vi "ESP301 Goto.vi"(5 "Axe Inv":bool, 6 "Input Units":i8(ring) items=["mm", "ps"], 7 "ESP301Ref":T1, 8 "error in":errorcluster, 9 "Axis":i8(ring)=1 items=["Axis 1"=1, "Axis 2"=2, "Axis 3"=3], 10 "Position":dbl=0.5, 11 "VISA Rsrc":refnum<visa-resource-name>="GPIB0::7::INSTR") -> (0 "error out":errorcluster, 1 "HighLim":bool, 2 "Pos Out":dbl=0.5, 3 "Warning":bool, 4 "LowLim":bool)   [LabVIEW 2019]
uses:
  <userlib>/ESP300/ESP300 GotoState.ctl
panel:
  out "Move Done":bool
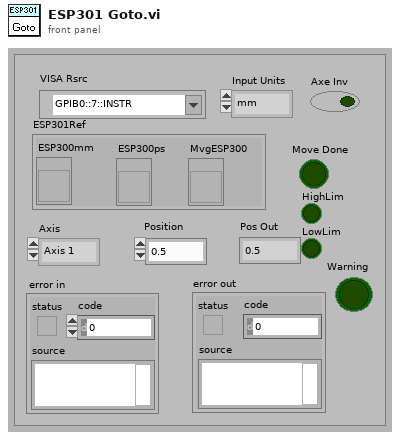
[diagram p1: front panel]
types:
  T1 = cluster{"ESP300mm":refnum<vi>, "ESP300ps":refnum<vi>, "MvgESP300":refnum<vi>}
  T2 = typedef "ESP300 GotoState.ctl" = enum16{"send command", "read position", "check status", "end"}
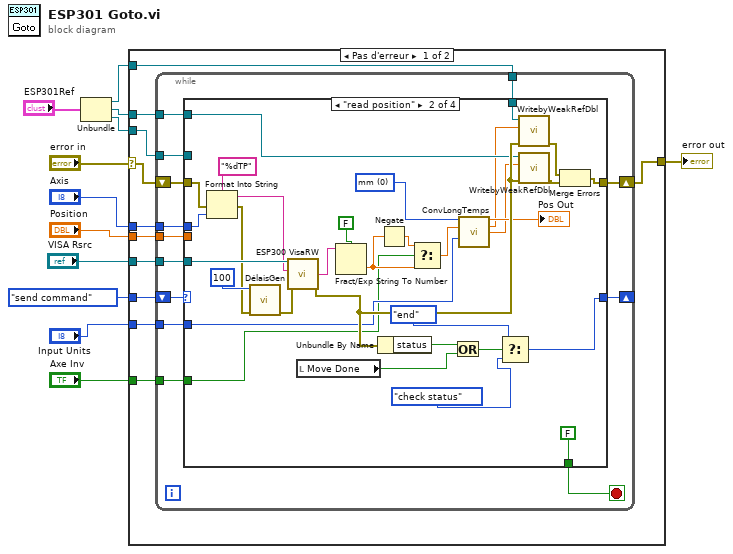
[diagram p0: block diagram]
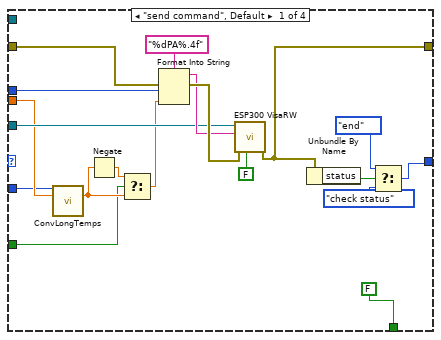
[diagram p2: hidden frame]
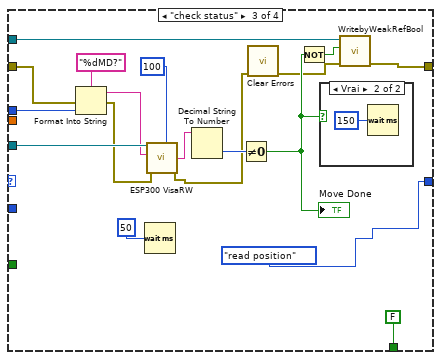
[diagram p3: hidden frame]
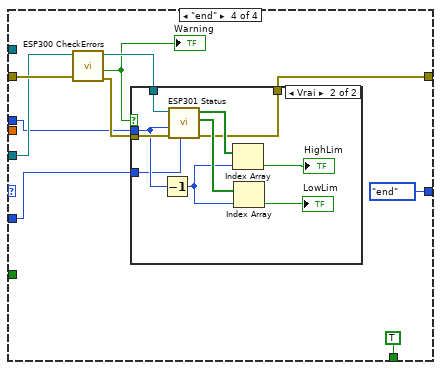
[diagram p5: hidden frame]
diagram:
  n1 = Unbundle("ESP301Ref") -> ("ESP300mm"=w2:refnum<vi>, "ESP300ps"=w4:refnum<vi>, "MvgESP300"=w3:refnum<vi>)
  n2 = case shown="Pas d'erreur" "error in" {
    selector: "error in" -> [w20 w128]
    tunnel: "Axis" -> [w22 _]
    tunnel: "Position" -> [w23 _]
    tunnel: [w19 w128] -> w9
    tunnel: ESP300_GotoState."send command" ("Énum") -> [w21 _]
    tunnel: "VISA Rsrc" -> [w18 _]
    tunnel: w3 -> [w17 _]
    tunnel: "Input Units" -> [w16 _]
    tunnel: w2 -> [w15 _]
    tunnel: w4 -> [w14 _]
    tunnel: "Axe Inv" -> [w13 _]
    frame No Error {
      n3 = while {
        tunnel: w23 -> [w36]
        tunnel: w22 -> [w35]
        shift-right: [w31] -> w19
        shift-left: w20 -> [w33]
        tunnel: w18 -> [w32]
        shift-right: [w29] -> _
        shift-left: w21 -> [w34]
        tunnel: w17 -> [w28]
        tunnel: w16 -> [w27]
        tunnel: w15 -> [w26]
        tunnel: w14 -> [w25]
        tunnel: w13 -> [w24]
        stop <- w30 stop-if-true
        n4 = case shown="\"read position\"" w34 {
          tunnel: w36 -> [w42 _ _ _]
          tunnel: w35 -> [w54 w85 w103 w108]
          tunnel: w33 -> [w53 w84 w102 w114]
          tunnel: w32 -> [w50 w87 w105 w113]
          tunnel: [w47 w68 w90 w109] -> w31
          tunnel: [FALSE FALSE FALSE TRUE] -> w30
          tunnel: [w44 w77 ESP300_GotoState."read position" ("Énum") ESP300_GotoState."end" ("Énum")] -> w29
          tunnel: w28 -> [_ _ w88 _]
          tunnel: w27 -> [w41 w60 _ w107]
          tunnel: w26 -> [_ w66 _ _]
          tunnel: w25 -> [_ w65 _ _]
          tunnel: w24 -> [w37 w56 _ _]
          frame "send command", Default {
            n5 = call <userlib>:"ConvLongTemps.vi"("Input Units"=w41, "Units Input"=w42) -> ("Units mm"=w38:dbl)  [unwired: 10 in, 3 out]
            n6 = Negate(x=w38) -> (-x=w39:dbl)
            n7 = Select(t=w39, s=w37, f=w38) -> (s? t:f=w40:dbl)
            n8 = Format Into String(format string="%dPA%.4f", error in=w53, w54, w40) -> (resulting string=w51:string, error out=w52:errorcluster)  [unwired: 1 in]
            n9 = call <userlib>:"ESP300 VisaRW.vi"("Lecture?(T)"=FALSE, "error in (no error)"=w52, "ChaineCom"=w51, "VISA Rsrc"=w50) -> ("error out"=w47:errorcluster)  [unwired: 3 in, 3 out]
            n10 = Unbundle By Name(w47) -> ("status"=w46:bool)
            n11 = Select(t=ESP300_GotoState."end" ("Énum"), s=w46, f=ESP300_GotoState."check status" ("Énum")) -> (s? t:f=w44:T2)
          }
          frame "read position" {
            w64 = i8 0 items=["mm", "ps"] ("Input Units")
            n12 = Format Into String(format string="%dTP", error in=w84, w85) -> (resulting string=w83:string, error out=w72:errorcluster)  [unwired: 1 in]
            n13 = call "DélaisGen.vi"("error in (no error)"=w72, "ms To Wait"=u32 100 ("milliseconds to wait")) -> ("error out"=w73:errorcluster)  [unwired: 9 in]
            n14 = call <userlib>:"ESP300 VisaRW.vi"("error in (no error)"=w73, "ChaineCom"=w83, "VISA Rsrc"=w87) -> ("error out"=w69:errorcluster, "ChaineRep"=w82:string)  [unwired: 4 in, 2 out]
            n15 = local read "Move Done"() -> (w71:bool)
            n16 = Fract/Exp String To Number(use system decimal point (T)=FALSE ("utiliser le séparateur décimal du système (V)"), string=w82) -> (number=w58:dbl)  [unwired: 2 in, 1 out]
            n17 = Unbundle By Name(w69) -> ("status"=w76:bool)
            n18 = Negate(x=w58) -> (-x=w59:dbl)
            n19 = Select(t=w59, s=w56, f=w58) -> (s? t:f=w57:dbl)
            n20 = Or(x=w76, y=w71) -> (x .or. y?=w75:bool)
            n21 = call <userlib>:"ConvLongTemps.vi"("Input Units"=w64, "Units Input"=w57, "Output Units"=w60) -> ("Units Output"=→"Pos Out":dbl, "Units mm"=w62:dbl, "Units ps"=w61:dbl)  [unwired: 9 in, 1 out]
            n22 = Select(t=ESP300_GotoState."end" ("Énum"), s=w75, f=ESP300_GotoState."check status" ("Énum")) -> (s? t:f=w77:T2)
            n23 = call <userlib>:"WritebyWeakRefDbl.vi"("error in"=w69, "Valeur"=w62, "Control Ref"=w66) -> ("error out"=w67:errorcluster)  [unwired: 8 in]
            n24 = call <userlib>:"WritebyWeakRefDbl.vi"("error in"=w69, "Valeur"=w61, "Control Ref"=w65) -> ("error out"=w70:errorcluster)  [unwired: 8 in]
            n25 = Merge Errors(w67, w70) -> (w68:errorcluster)
          }
          frame "check status" {
            n26 = Format Into String(format string="%dMD?", error in=w102, w103) -> (resulting string=w100:string, error out=w101:errorcluster)  [unwired: 1 in]
            n27 = Wait (ms)(milliseconds to wait=u32 50 ("attente (ms)")) -> ()  [unwired: 1 out]
            n28 = call <userlib>:"ESP300 VisaRW.vi"("Délais (0 ms)"=u32 100, "error in (no error)"=w101, "ChaineCom"=w100, "VISA Rsrc"=w105) -> ("error out"=w95:errorcluster, "ChaineRep"=w99:string)  [unwired: 3 in, 2 out]
            n29 = Decimal String To Number(string=w99) -> (number=w97:i32)  [unwired: 2 in, 1 out]
            n30 = Not Equal To 0?(x=w97) -> (x != 0?=w94:bool)
            "Move Done" <- w94
            n31 = call <vilib>:"Clear Errors.vi"("error in (no error)"=w95) -> ("error out"=w91:errorcluster)  [unwired: 5 in, 1 out]
            n32 = Not(x=w94) -> (.not. x?=w89:bool)
            n33 = case shown="Vrai" w94 {
              frame False {
              }
              frame True {
                n34 = Wait (ms)(milliseconds to wait=u32 150) -> ()  [unwired: 1 out]
              }
            }
            n35 = call <userlib>:"WritebyWeakRefBool.vi"("error in"=w91, "Valeur"=w89, "Control Ref"=w88) -> ("error out"=w90:errorcluster)  [unwired: 8 in]
          }
          frame "end" {
            n36 = call <userlib>:"ESP300 CheckErrors.vi"("error in (no error)"=w114, "Ressource VISA In"=w113) -> ("error out"=w110:errorcluster, "Warning"=w111:bool, "Ressource VISA Out"=w112:refnum<visa-resource-name>)  [unwired: 4 in, 1 out]
            "Warning" <- w111
            n37 = case shown="Vrai" w111 {
              tunnel: w112 -> [_ w127]
              tunnel: w110 -> [w117 w124]
              tunnel: [w117 w123] -> w109
              tunnel: w108 -> [_ w122]
              tunnel: w107 -> [_ w120]
              frame False {
              }
              frame True {
                n38 = Decrement(x=w122) -> (x-1=w121:i8)
                n39 = call <userlib>:"ESP301 Status.vi"("Input Units"=w120, "error in"=w124, "Axis"=w122, "VISA Rsrc"=w127) -> ("error out"=w123:errorcluster, "Low Limit"=w125:bool[], "High Limit"=w126:bool[])  [unwired: 4 in, 1 out]
                n40 = Index Array(array=w126, index=w121) -> (element=→"HighLim":bool)
                n41 = Index Array(array=w125, index=w121) -> (element=→"LowLim":bool)
              }
            }
          }
        }
      }
    }
    frame Error {
    }
  }
  "error out" <- w9
